vi "Get Max Profile Size.vi"() -> (1 "Profile Size":u32)   [LabVIEW 2015, in "KEYENCE LJ-X8000A.lvlib"]
uses:
  KEYENCE LJ-X8000A.lvlib
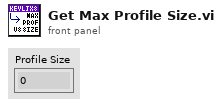
[diagram p1: front panel]
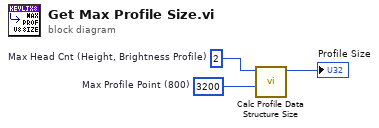
[diagram p0: block diagram]
diagram:
  w2 = u16 3200  # Max Profile Point (800)
  w3 = u8 2  # Max Head Cnt (Height, Brightness Profile)
  n1 = call "Calc Profile Data Structure Size.vi"("Profile Data Point"=w2, "Profile Cnt"=w3) -> ("Profile Size(Byte)"=→"Profile Size":u32)  [unwired: 8 in, 1 out]
